vi "Config - Read.vi"(8 "error in (no error)":errorcluster, 11 "View Model":T1) -> (0 "error out":errorcluster, 3 "View Model":T1)   [LabVIEW 2017]
doc: "Reads DB record from Configuration database."
uses:
  View Model/Controls/View Model.ctl
  View Model/Controls/Shared Model.ctl
  Error/Controls/Error Model.ctl
  Error/Controls/Error Event.ctl
  Error/Controls/Error Type.ctl
  Controls/Config DB Model.ctl
  Controls/Config DB Command.ctl
  Controls/Config DB Record.ctl
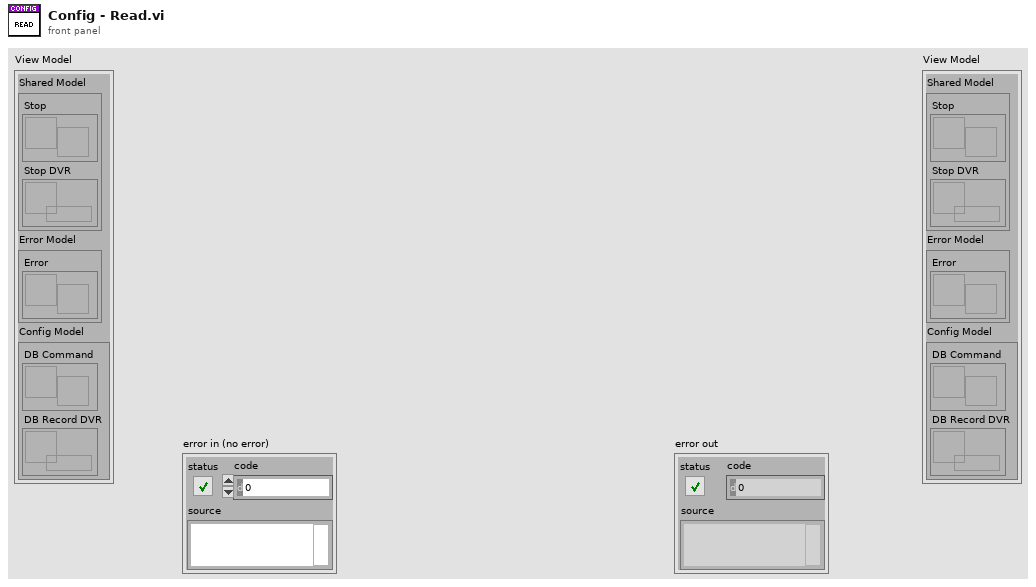
[diagram p1: front panel]
types:
  T1 = typedef "View Model.ctl" = cluster{"Shared Model":T2, "Error Model":T3, "Config Model":T4}
  T2 = typedef "Shared Model.ctl" = cluster{"Stop":refnum<user-event>, "Stop DVR":refnum<data-value>}
  T3 = typedef "Error Model.ctl" = cluster{"Error":refnum<user-event>}
  T4 = typedef "Config DB Model.ctl" = cluster{"DB Command":refnum<user-event>, "DB Record DVR":refnum<data-value>}
  T5 = typedef "Config DB Record.ctl" = cluster{"Door Open":dbl, "Door Close":dbl, "Travel Time":dbl, "Inactivity Time":dbl}
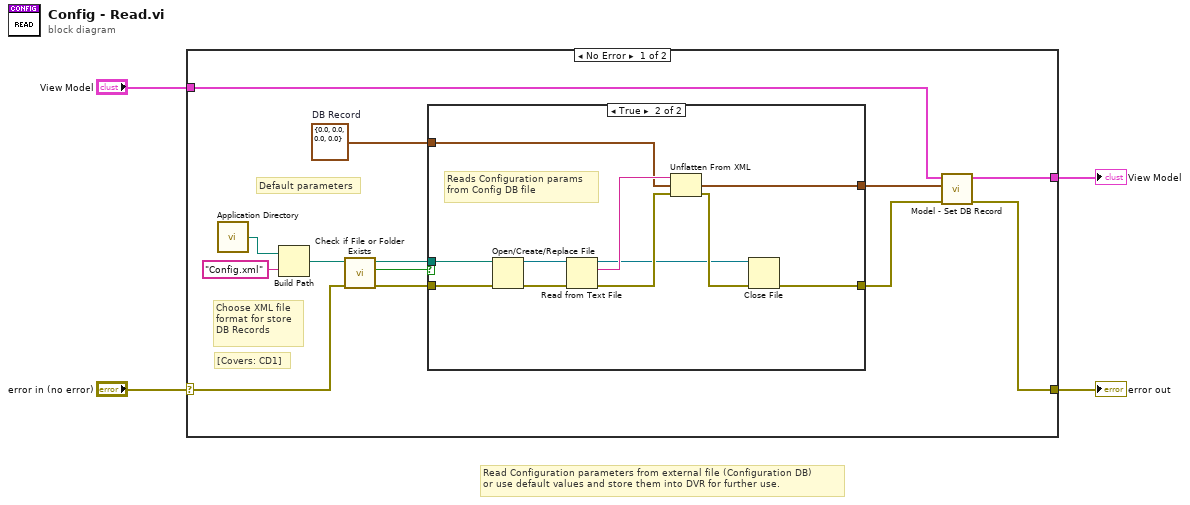
[diagram p0: block diagram]
diagram:
  # "Read Configuration parameters from external file (Configuration DB)\nor use default values and store them into DVR for further use."
  n1 = case shown="No Error" "error in (no error)" {
    selector: "error in (no error)" -> [w14 w31]
    tunnel: "View Model" -> [w5 w32]
    tunnel: [w6 w32] -> w2
    tunnel: [w7 w31] -> w1
    frame No Error {
      w10 = T5 {"Door Open"=0.0, "Door Close"=0.0, "Travel Time"=0.0, "Inactivity Time"=0.0}  # DB Record
      # "Default parameters"
      # "[Covers: CD1]"
      # "Choose XML file\nformat for store\nDB Records"
      n2 = call <vilib>:"Application Directory.vi"() -> ("Application Directory"=w17:path)
      n3 = Build Path(base path=w17, name or relative path="Config.xml") -> (appended path=w15:path)
      n4 = call <vilib>:"Check if File or Folder Exists.vi"("error in (no error)"=w14, "path"=w15) -> ("error out"=w11:errorcluster, "file or folder exists?"=w13:bool, "dup path"=w12:path)  [unwired: 7 in]
      n5 = case shown="True" w13 {
        tunnel: w12 -> [_ w29]
        tunnel: w11 -> [w18 w30]
        tunnel: w10 -> [w19 w25]
        tunnel: [w19 w21] -> w9
        tunnel: [w18 w20] -> w8
        frame False {
          # "[Covers: CD3]"
          # "If Configuration DB is not found\nuse default parameters"
        }
        frame True {
          # "Reads Configuration params\nfrom Config DB file"
          n6 = Open/Create/Replace File(file path (use dialog)=w29, error in=w30) -> (refnum out=w27:refnum<file>, error out=w28:errorcluster)  [unwired: 4 in, 1 out]
          n7 = Read from Text File(file (use dialog)=w27, error in=w28) -> (refnum out=w22:refnum<file>, text=w26:string, error out=w24:errorcluster)  [unwired: 2 in, 1 out]
          n8 = Unflatten From XML(xml string=w26, type=w25, error in (no error)=w24) -> (value=w21:T5, error out=w23:errorcluster)
          n9 = Close File(refnum=w22, error in=w23) -> (error out=w20:errorcluster)  [unwired: 1 out]
        }
      }
      n10 = call "Model - Set DB Record.vi"("error in (no error)"=w8, "DB Record"=w9, "View Model"=w5) -> ("error out"=w7:errorcluster, "View Model"=w6:T1)  [unwired: 7 in]
    }
    frame Error {
    }
  }
  "error out" <- w1
  "View Model" <- w2
